vi "Match.vi"(10 "log record":T1 {"timestamp" format="%<%x %.3X>T"}, 11 "data item":refnum<class "Data Item.lvclass">) -> (2 "matches":bool[](array[boolean]), 3 "dup data item":refnum<class "Data Item.lvclass">)   [LabVIEW 2018, in "Logging.lvlib" / "Data Item.lvclass"]
uses:
  Data Item.lvclass
  Log Record.ctl
  Logger/Internal Log Levels.ctl
  Data Item.lvclass/Data Item.ctl
  <vilib>/Utility/Data Type/NI_Data Type.lvlib
  Logging.lvlib
panel:
  # "Connector Pane"
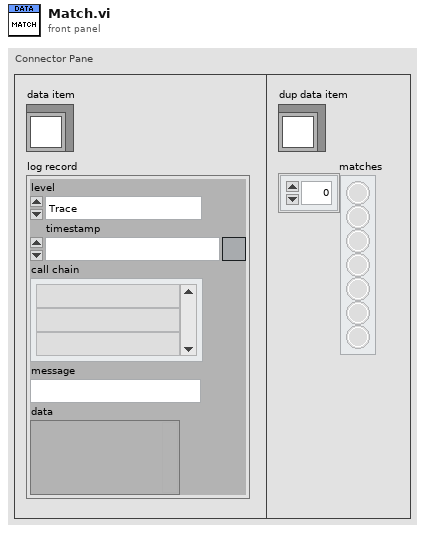
[diagram p1: front panel]
types:
  T1 = typedef "Logging.lvlib/Log Record.ctl" = cluster{"level":T2, "timestamp":timestamp, "call chain":string[], "message":string, "data":variant}
  T2 = typedef "Logging.lvlib/Internal Log Levels.ctl" = enum16{"Trace", "Debug", "Info", "Warning", "Error", "Critical", "Internal"}
  T3 = typedef "NI_Data Type.lvlib/Data Type.ctl" = enum8{"Invalid Type", "Void", "I8", "I16", "I32", "I64", "U8", "U16", "U32", "U64", "Single Float", "Double Float", "Extended Float", "Single Complex", "Double Complex", "Extended Complex", "Enum U8", "Enum U16", "Enum U32", "Enum U64", "Single Float With Unit", "Double Float With Unit", "Extended Float With Unit", "Single Complex with Unit", "Double Complex with Unit", "Extended Complex with Unit", "Boolean", "String", "Path", "Picture", "Tag", "Array", "Cluster", "Variant", "LV Variant", "Waveform", "Timestamp", "Digital Waveform", "Digital Data", "ExpressData", "Refnum", "External Data", "VI", "Poly VI", "LabVIEW Class Instance", "Fixed Point", "Set Collection", "Map Collection"}
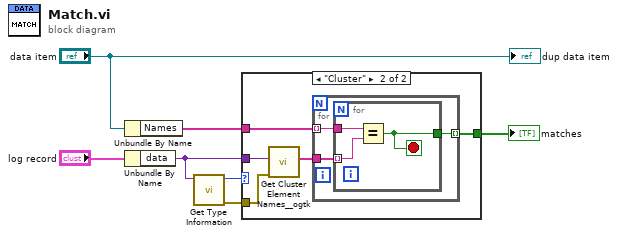
[diagram p0: block diagram]
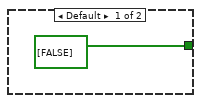
[diagram p2: hidden frame]
diagram:
  n1 = Unbundle By Name("data item") -> ("Names"=w5:string[])
  n2 = Unbundle By Name("log record") -> ("data"=w4:variant)
  n3 = call <vilib>:"Get Type Information.vi"("variant"=w4) -> ("error out"=w3:errorcluster, "type"=w6:T3)  [unwired: 6 in, 3 out]
  n4 = case shown="\"Cluster\"" w6 {
    tunnel: w5 -> [_ w11]
    tunnel: [bool[] [FALSE] w9] -> w1
    tunnel: w4 -> [_ w13]
    tunnel: w3 -> [_ w10]
    frame Default {
    }
    frame "Cluster" {
      n5 = call <userlib>:"Get Cluster Element Names__ogtk.vi"("error in (no error)"=w10, "Cluster"=w13) -> ("Element Names"=w12:string[])  [unwired: 8 in, 1 out]
      n6 = for {
        tunnel: w12 -> [w15]
        tunnel: w11 -> [w16] mode=indexing
        tunnel: [w14] -> w9 mode=indexing
        n7 = for {
          tunnel: w16 -> [w19]
          tunnel: w15 -> [w18] mode=indexing
          tunnel: [w17] -> w14
          stop <- w17 stop-if-true
          n8 = Equal?(x=w19, y=w18) -> (x = y?=w17:bool)
        }
      }
    }
  }
  "matches" <- w1
  "dup data item" <- "data item"
